vi "Index_Logic.vi"(0 "X":bool, 4 "Intake Pressed":bool, 6 "B":bool, 7 "Right Trigger":dbl, 8 "Y":bool, 9 "A":bool, 10 "Reject Pressed":bool, 11 "Elevate Pressed":bool) -> ()   [LabVIEW 2020]
uses:
  <vilib>/Rock Robotics/WPI/ThirdParty/Phoenix-LabVIEW/Motor Controller/Controls/CTRE_Phoenix_MotorControl_ControlMode.ctl
  <vilib>/Rock Robotics/WPI/Solenoid/WPI_SolenoidValue.ctl
  <vilib>/Rock Robotics/Network Tables/NT Read String.vi
  <vilib>/Rock Robotics/Network Tables/NT Write Boolean.vi
  <vilib>/Rock Robotics/WPI/Solenoid/WPI_SolenoidSetEnum.vi
  <vilib>/Rock Robotics/Network Tables/NT Write Number.vi
panel:
  in  "Intake want":dbl=0.75
  in  "Elevate want":dbl=-0.35
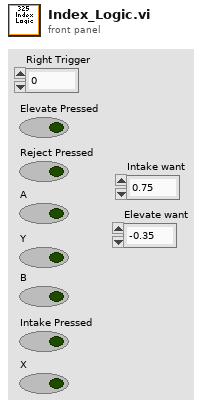
[diagram p1: front panel]
types:
  T1 = typedef "CTRE_Phoenix_MotorControl_ControlMode.ctl" = u16
  T2 = typedef "WPI_SolenoidValue.ctl" = enum16{"Off", "On", "Forward", "Reverse"}
  T3 = typedef "WPI_SolenoidDevRef.ctl" = cluster{"DevStatus":errorcluster, "Pneumatics Control Module":u8, "Forward Solenoid Channel":T4, "Reverse Solenoid Channel":T4}
  T4 = typedef "WPI_SolenoidChannel.ctl" = enum8{"Solenoid 0", "Solenoid 1", "Solenoid 2", "Solenoid 3", "Solenoid 4", "Solenoid 5", "Solenoid 6", "Solenoid 7", "Solenoid 8", "Solenoid 9", "Solenoid 10", "Solenoid 11", "Solenoid 12", "Solenoid 13", "Solenoid 14", "Solenoid 15", "Invalid"}
  T5 = typedef "WPI_MotorControlDeviceRef.ctl" = cluster{"DeviceStatus":errorcluster, "Type":T6, "PWM":cluster{"PWM Channel":T7, "DeadBand":T8}, "CAN":cluster{"Device Number":u8, "SetOutput VI Ref":variant, "GetOutput VI Ref":variant, "Enable VI Ref":variant, "Disable VI Ref":variant, "Data":variant}, "Invert":bool, "DIO PWM":cluster{"PWM \"Enable\" Channel":T7, "DIOChannel":T9, "PWM Rate":dbl}}
  T6 = typedef "WPI_MotorControlType.ctl" = enum16{"PWM", "CAN", "DIO PWM"}
  T7 = typedef "FPGA_DIOPWMChannel.ctl" = enum8{"PWM 0", "PWM 1", "PWM 2", "PWM 3", "PWM 4", "PWM 5", "PWM 6", "PWM 7", "PWM 8", "PWM 9", "PWM MXP 0", "PWM MXP 1", "PWM MXP 2", "PWM MXP 3", "PWM MXP 4", "PWM MXP 5", "PWM MXP 6", "PWM MXP 7", "PWM MXP 8", "PWM MXP 9", "Invalid"}
  T8 = typedef "WPI_PWMDeadband.ctl" = cluster{"Name":string, "maxPositivePwm":i32, "minPositivePwm":i32, "centerPwm":i32, "maxNegativePwm":i32, "minNegativePwm":i32, "angularRange":u16}
  T9 = typedef "FPGA_DIOChannel.ctl" = enum8{"DIO 0", "DIO 1", "DIO 2", "DIO 3", "DIO 4", "DIO 5", "DIO 6", "DIO 7", "DIO 8", "DIO 9", "DIO MXP 0", "DIO MXP 1", "DIO MXP 2", "DIO MXP 3", "DIO MXP 4", "DIO MXP 5", "DIO MXP 6", "DIO MXP 7", "DIO MXP 8", "DIO MXP 9", "DIO MXP 10", "DIO MXP 11", "DIO MXP 12", "DIO MXP 13", "DIO MXP 14", "DIO MXP 15", "SPI Port CS1", "SPI Port CS2", "SPI Port CS3", "SPI Port MISO", "SPI Port MOSI", "Invalid"}
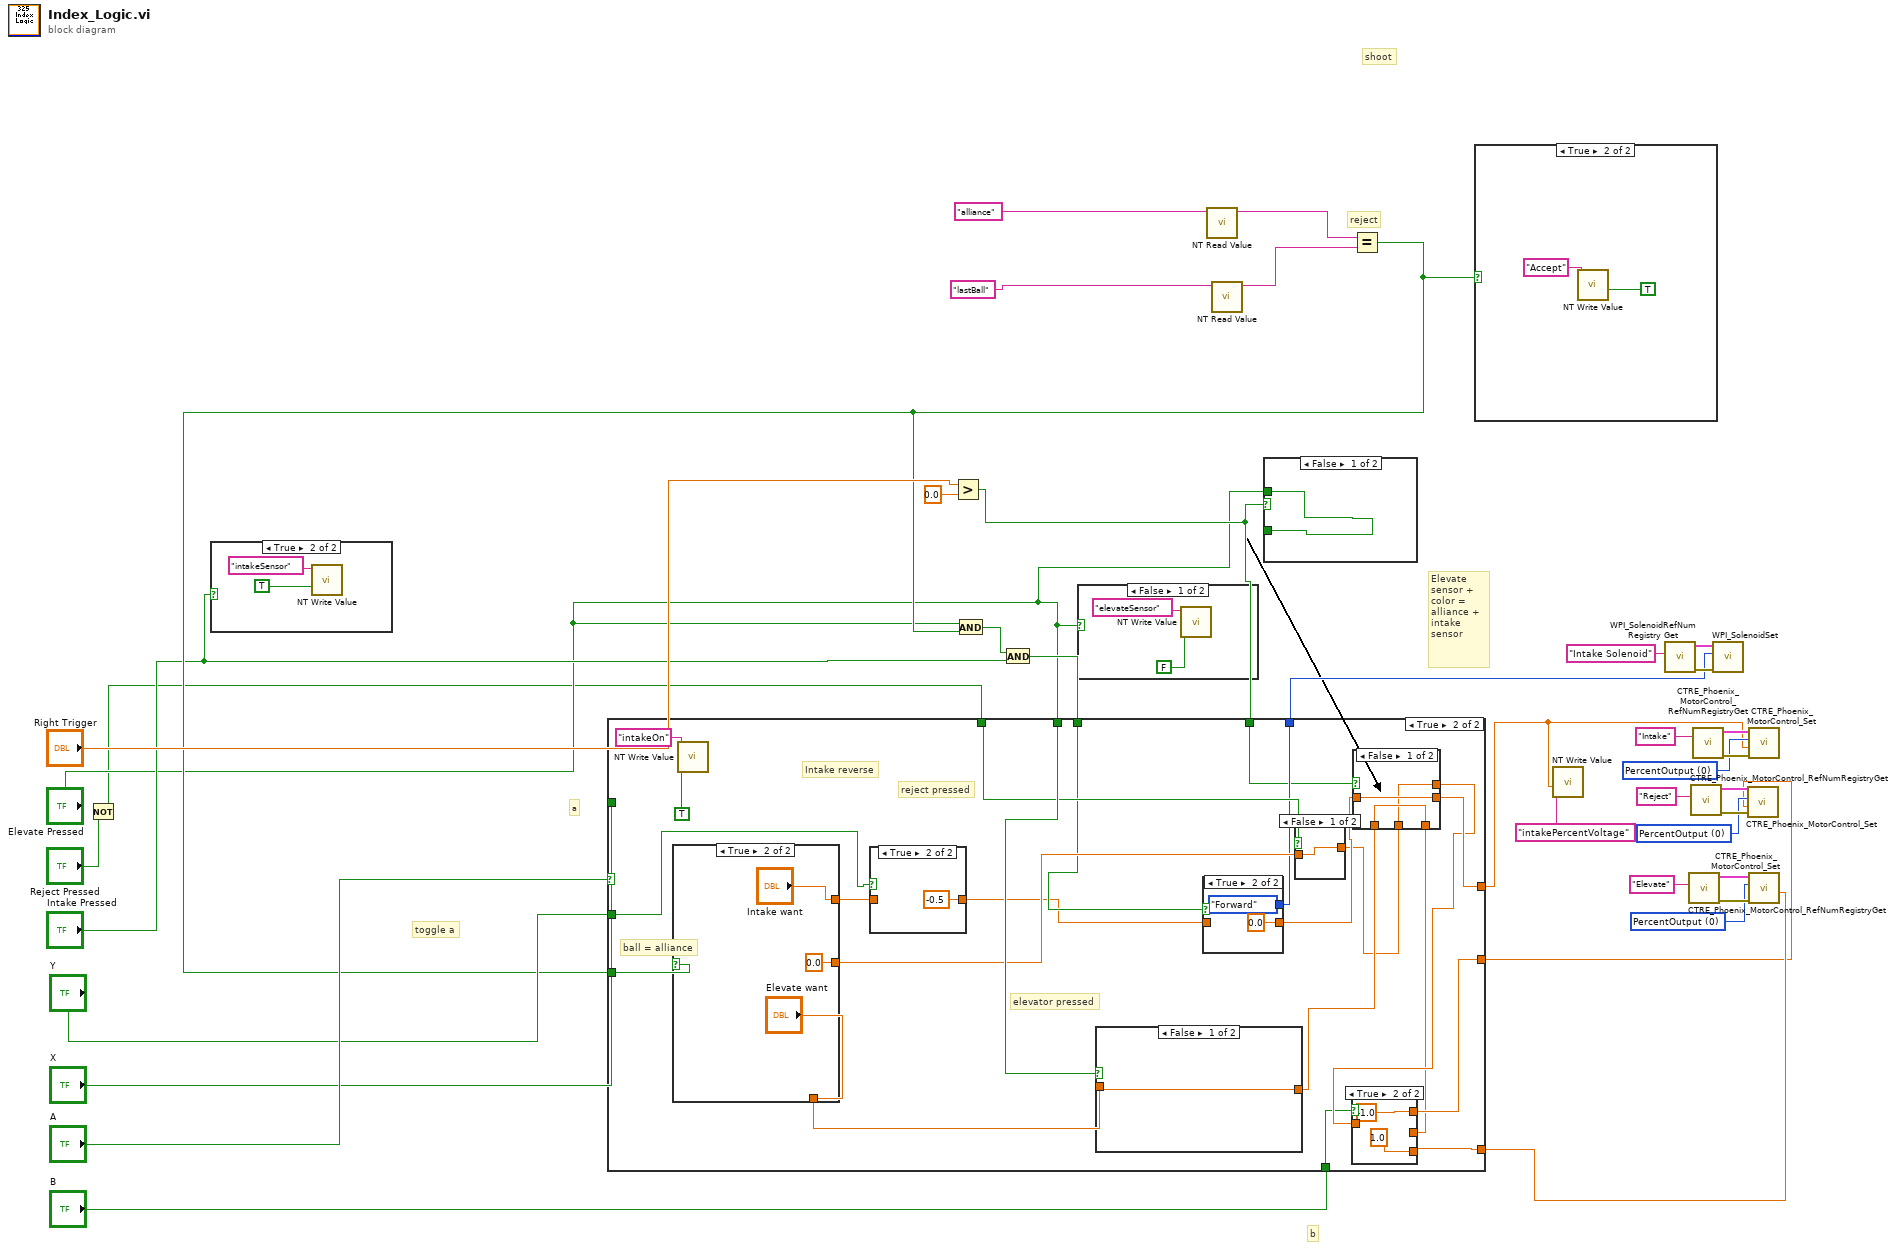
[diagram p0: block diagram]
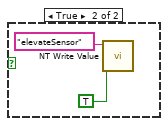
[diagram p2: hidden frame]
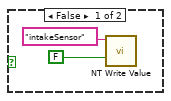
[diagram p3: hidden frame]
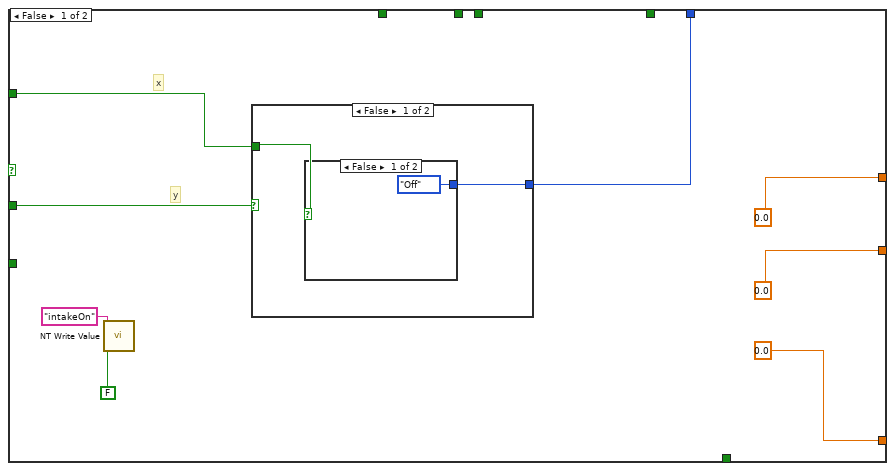
[diagram p4: hidden frame]
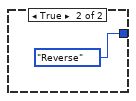
[diagram p5: hidden frame]
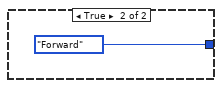
[diagram p6: hidden frame]
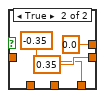
[diagram p9: hidden frame]
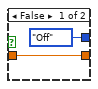
[diagram p10: hidden frame]
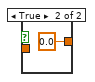
[diagram p11: hidden frame]
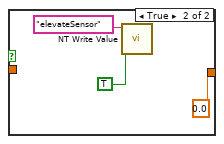
[diagram p12: hidden frame]
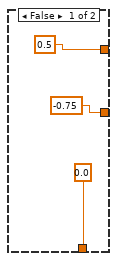
[diagram p13: hidden frame]
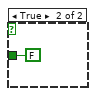
[diagram p14: hidden frame]
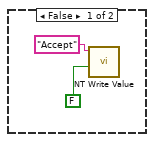
[diagram p15: hidden frame]
diagram:
  w27 = T1 0 items=["PercentOutput"=0, "Position"=1, "Velocity"=2, "Current"=3, "Follower"=5, "MotionProfile"=6, "MotionMagic"=7, "MotionProfileArc"=10, "Disabled"=15] ("Control Mode")
  w28 = T1 0 items=["PercentOutput"=0, "Position"=1, "Velocity"=2, "Current"=3, "Follower"=5, "MotionProfile"=6, "MotionMagic"=7, "MotionProfileArc"=10, "Disabled"=15] ("Control Mode")
  w29 = T1 0 items=["PercentOutput"=0, "Position"=1, "Velocity"=2, "Current"=3, "Follower"=5, "MotionProfile"=6, "MotionMagic"=7, "MotionProfileArc"=10, "Disabled"=15] ("Control Mode")
  # "toggle a"
  # "Elevate sensor + color = alliance + intake sensor"
  # "b"
  # "a"
  # "shoot"
  # "reject"
  n1 = Not(x="Reject Pressed") -> (.not. x?=w2:bool)
  n2 = case shown="True" "Intake Pressed" {
    frame False {
      n3 = call-poly <vilib>:"NT Write Value.vi"("Boolean"=FALSE, "Name"="intakeSensor") -> ()  [unwired: 9 in, 1 out]
    }
    frame True {
      n4 = call-poly <vilib>:"NT Write Value.vi"("Boolean"=TRUE, "Name"="intakeSensor") -> ()  [unwired: 9 in, 1 out]
    }
  }
  n5 = Greater?(x="Right Trigger", y=0.0) -> (0:w13:bool)
  n6 = case shown="False" "Elevate Pressed" {
    frame False {
      n7 = call-poly <vilib>:"NT Write Value.vi"("Boolean"=FALSE, "Name"="elevateSensor") -> ()  [unwired: 9 in, 1 out]
    }
    frame True {
      n8 = call-poly <vilib>:"NT Write Value.vi"("Boolean"=TRUE, "Name"="elevateSensor") -> ()  [unwired: 9 in, 1 out]
    }
  }
  n9 = call-poly <vilib>:"NT Read Value.vi"("Name"="alliance") -> ("String"=w26:string)  [unwired: 9 in, 1 out]
  n10 = call-poly <vilib>:"NT Read Value.vi"("Name"="lastBall") -> ("String"=w23:string)  [unwired: 9 in, 1 out]
  n11 = case shown="False" w13 {
    tunnel: "Elevate Pressed" -> [w47 _]
    tunnel: [w47 FALSE ("Switch Pressed")] -> _
    frame False {
    }
    frame True {
    }
  }
  n12 = Equal?(x=w26, y=w23) -> (x = y?=w6:bool)
  n13 = And(x="Elevate Pressed", y=w6) -> (x .and. y?=w17:bool)
  n14 = And(x=w17, y="Intake Pressed") -> (x .and. y?=w16:bool)
  n15 = case shown="True" "A" {
    tunnel: w6 -> [_ w83]
    tunnel: [0.0 ("Intake want") w76] -> w1
    tunnel: [0.0 ("Elevate 1") w68] -> w19
    tunnel: "Elevate Pressed" -> [_ w82]
    tunnel: [0.0 ("Reject no want") w71] -> w18
    tunnel: w2 -> [_ w80]
    tunnel: w16 -> [_ w67]
    tunnel: [w53 w78] -> w15
    tunnel: w13 -> [_ w74]
    tunnel: "B" -> [_ w70]
    tunnel: "Y" -> [w52 w66]
    tunnel: "X" -> [w51 _]
    frame False {
      # "x"
      # "y"
      n16 = call-poly <vilib>:"NT Write Value.vi"("Boolean"=FALSE, "Name"="intakeOn") -> ()  [unwired: 9 in, 1 out]
      n17 = case shown="False" w52 {
        tunnel: [w58 WPI_SolenoidValue."Forward" ("Value")] -> w53
        tunnel: w51 -> [w57 _]
        frame False {
          n18 = case shown="False" w57 {
            tunnel: [WPI_SolenoidValue."Off" ("Value") WPI_SolenoidValue."Reverse" ("Value")] -> w58
            frame False {
            }
            frame True {
            }
          }
        }
        frame True {
        }
      }
    }
    frame True {
      # "Intake reverse"
      # "reject pressed"
      # "elevator pressed"
      # "ball = alliance"
      n19 = case shown="True" w83 {
        tunnel: [0.0 ("Elevate want") "Elevate want"] -> w81
        tunnel: [0.5 ("Intake 1") "Intake want"] -> w64
        tunnel: [-0.75 ("Reject no want") 0.0 ("Reject no want")] -> w79
        frame False {
        }
        frame True {
        }
      }
      n20 = call-poly <vilib>:"NT Write Value.vi"("Boolean"=TRUE, "Name"="intakeOn") -> ()  [unwired: 9 in, 1 out]
      n21 = case shown="True" w66 {
        tunnel: [w84 -0.5 ("Intake want")] -> w65
        tunnel: w64 -> [w84 _]
        frame False {
        }
        frame True {
        }
      }
      n22 = case shown="False" w82 {
        tunnel: [w102 0.0 ("Elevate 1")] -> w75
        tunnel: w81 -> [w102 _]
        frame False {
        }
        frame True {
          n23 = call-poly <vilib>:"NT Write Value.vi"("Boolean"=TRUE, "Name"="elevateSensor") -> ()  [unwired: 9 in, 1 out]
        }
      }
      n24 = case shown="True" w67 {
        tunnel: w65 -> [w97 _]
        tunnel: [w97 0.0 ("Intake want")] -> w77
        tunnel: [WPI_SolenoidValue."Off" ("Value") WPI_SolenoidValue."Forward" ("Value")] -> w78
        frame False {
        }
        frame True {
        }
      }
      n25 = case shown="False" w80 {
        tunnel: w79 -> [w100 _]
        tunnel: [w100 0.0 ("Reject no want")] -> w73
        frame False {
        }
        frame True {
        }
      }
      n26 = case shown="False" w74 {
        tunnel: w77 -> [w92 _]
        tunnel: [w92 0.35 ("Intake want")] -> w76
        tunnel: w75 -> [w91 _]
        tunnel: [w91 -0.35 ("Elevate 1")] -> w69
        tunnel: w73 -> [w90 _]
        tunnel: [w90 0.0 ("Reject no want")] -> w72
        frame False {
        }
        frame True {
        }
      }
      n27 = case shown="True" w70 {
        tunnel: w72 -> [w87 _]
        tunnel: [w87 -1.0 ("Reject no want")] -> w71
        tunnel: w69 -> [w86 _]
        tunnel: [w86 1.0 ("Elevate 1")] -> w68
        frame False {
        }
        frame True {
        }
      }
    }
  }
  n28 = case shown="True" w6 {
    frame False {
      n29 = call-poly <vilib>:"NT Write Value.vi"("Boolean"=FALSE, "Name"="Accept") -> ()  [unwired: 9 in, 1 out]
    }
    frame True {
      n30 = call-poly <vilib>:"NT Write Value.vi"("Boolean"=TRUE, "Name"="Accept") -> ()  [unwired: 9 in, 1 out]
    }
  }
  n31 = call-poly <vilib>:"NT Write Value.vi"("Numeric"=w1, "Name"="intakePercentVoltage") -> ()  [unwired: 9 in, 1 out]
  n32 = call <vilib>:"WPI_SolenoidRefNum Registry Get.vi"("refnum name"="Intake Solenoid") -> ("error out"=w22:errorcluster, "SolenoidDevRef"=w21:T3)  [unwired: 9 in]
  n33 = call <vilib>:"CTRE_Phoenix_MotorControl_RefNumRegistryGet.vi"("refnum name"="Elevate") -> ("error out"=w34:errorcluster, "PhoenixMotorControlDevRef"=w33:T5)  [unwired: 9 in]
  n34 = call <vilib>:"CTRE_Phoenix_MotorControl_RefNumRegistryGet.vi"("refnum name"="Reject") -> ("error out"=w36:errorcluster, "PhoenixMotorControlDevRef"=w35:T5)  [unwired: 9 in]
  n35 = call <vilib>:"CTRE_Phoenix_MotorControl_RefNumRegistryGet.vi"("refnum name"="Intake") -> ("error out"=w38:errorcluster, "PhoenixMotorControlDevRef"=w37:T5)  [unwired: 9 in]
  n36 = call-poly <vilib>:"WPI_SolenoidSet.vi"("error in (no error)"=w22, "Value"=w15, "SolenoidDevRef"=w21) -> ()  [unwired: 7 in, 2 out]
  n37 = call <vilib>:"CTRE_Phoenix_MotorControl_Set.vi"("error in (no error)"=w36, "Output"=w18, "Control Mode"=w27, "PhoenixMotorControlDevRef"=w35) -> ()  [unwired: 6 in, 2 out]
  n38 = call <vilib>:"CTRE_Phoenix_MotorControl_Set.vi"("error in (no error)"=w38, "Output"=w1, "Control Mode"=w28, "PhoenixMotorControlDevRef"=w37) -> ()  [unwired: 6 in, 2 out]
  n39 = call <vilib>:"CTRE_Phoenix_MotorControl_Set.vi"("error in (no error)"=w34, "Output"=w19, "Control Mode"=w29, "PhoenixMotorControlDevRef"=w33) -> ()  [unwired: 6 in, 2 out]
